vi "FTW-Time-Display-Timestamp.vi"(3 "Format":T1, 4 "Timestamp (unwired for current time)":timestamp format="%^<%Y-%m-%dT%H:%M:%S%3uZ>T") -> (0 "Formatted Timestamp":string)   [LabVIEW 2013]
uses:
  FTW-Time-DisplayFormat-Timestamp.ctl
panel:
  # "Inputs"
  # "Outputs"
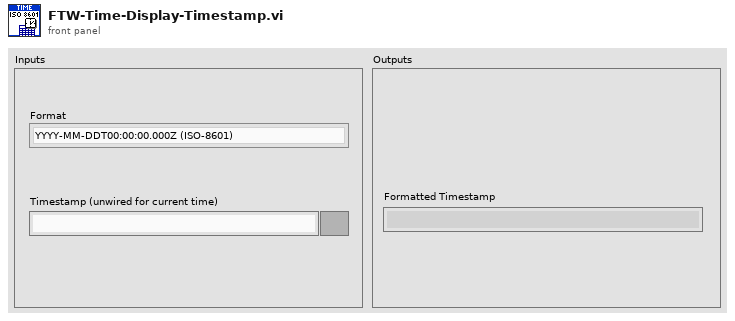
[diagram p1: front panel]
types:
  T1 = typedef "FTW-Time-DisplayFormat-Timestamp.ctl" = enum16{"YYYY-MM-DDT00:00:00.000Z (ISO-8601)", "YYYY-MM-DDT00-00-00Z (Simple ISO-8601)", "YYYY-MM-DD"}
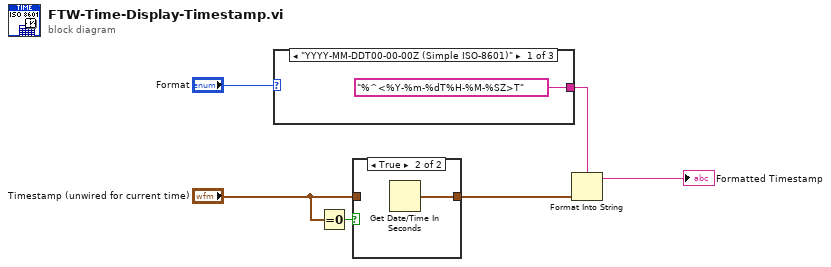
[diagram p0: block diagram]
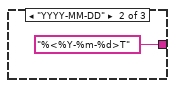
[diagram p2: hidden frame]
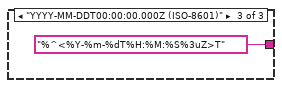
[diagram p3: hidden frame]
diagram:
  n1 = case shown="\"YYYY-MM-DDT00-00-00Z (Simple ISO-8601)\"" "Format" {
    tunnel: ["%^<%Y-%m-%dT%H-%M-%SZ>T" ("format string") "%<%Y-%m-%d>T" ("format string") "%^<%Y-%m-%dT%H:%M:%S%3uZ>T" ("format string")] -> w6
    frame "YYYY-MM-DDT00-00-00Z (Simple ISO-8601)" {
    }
    frame "YYYY-MM-DD" {
    }
    frame "YYYY-MM-DDT00:00:00.000Z (ISO-8601)" {
    }
  }
  n2 = Equal To 0?(x="Timestamp (unwired for current time)") -> (x = 0?=w4:bool)
  n3 = case shown="True" w4 {
    tunnel: [w10 w11] -> w5
    tunnel: "Timestamp (unwired for current time)" -> [w10 _]
    frame False {
    }
    frame True {
      n4 = Get Date/Time In Seconds() -> (seconds since 1Jan1904=w11:timestamp)
    }
  }
  n5 = Format Into String(format string=w6, w5) -> (resulting string=→"Formatted Timestamp":string)  [unwired: 2 in, 1 out]
